vi "Align Traces.vi"(0 "Data Input":T2(array[cluster]) {"Data Channels" format="%.2f"}, 1 "Alignment":enum16{"Vertically", "Horizontally"}(ring)=enum."Horizontally", 3 "Aligning Channel":i32, 4 "Y Level":dbl format="%.2f", 5 "X Level":dbl format="%.2f", 9 "Channels / Subject (in)":T1(array[cluster])=[[{"Start"=0, "End"=1000000, "Offset"=0.0, "Deleted"=FALSE}]] {"Offset" format="%.2f"}) -> (11 "Channels / Subject (out)":T1(array[cluster])=[[{"Start"=0, "End"=1000000, "Offset"=0.0, "Deleted"=FALSE}]] {"Offset" format="%.2f"})   [LabVIEW 2013, in "impulse functions.lvlib"]
uses:
  impulse functions.lvlib
panel:
  # "Copyright Americo A. Migliaccio (c) 2002 All Rights Reserved by Author"
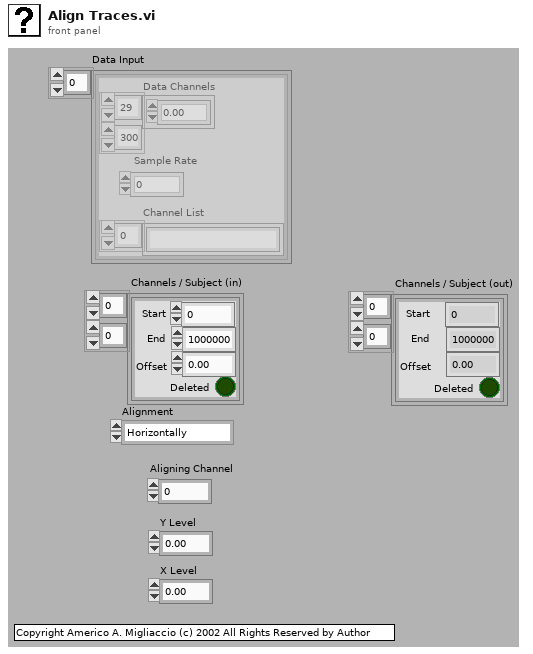
[diagram p1: front panel]
types:
  T1 = cluster{"Start":i32, "End":i32, "Offset":dbl, "Deleted":bool}[][]
  T2 = cluster{"Data Channels":dbl[][], "Sample Rate":i32, "Channel List":string[]}[]
  T3 = cluster{"Start":i32, "End":i32, "Offset":dbl, "Deleted":bool}
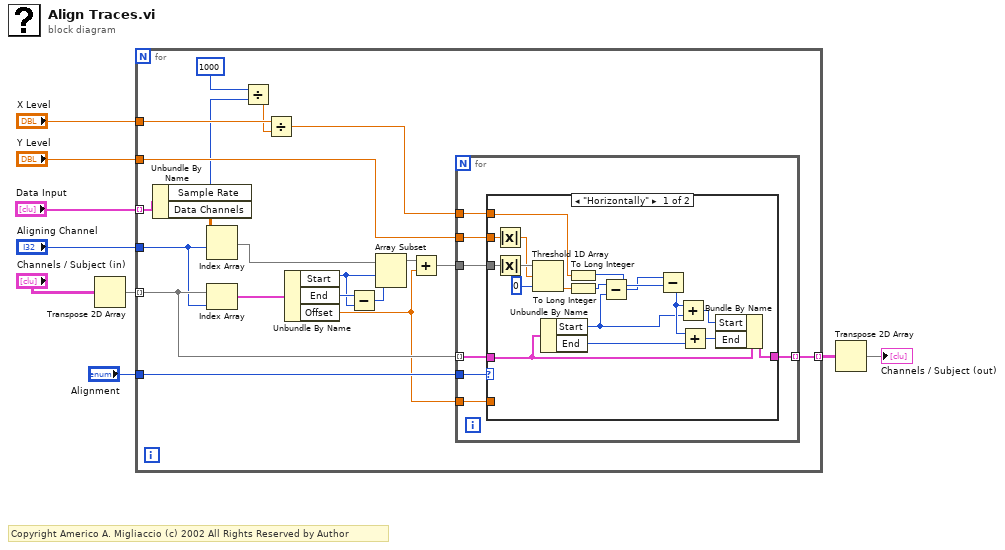
[diagram p0: block diagram]
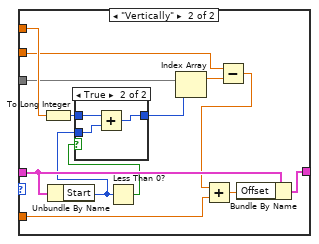
[diagram p2: hidden frame]
diagram:
  # "Copyright Americo A. Migliaccio (c) 2002 All Rights Reserved by Author"
  n1 = Transpose 2D Array(2D array="Channels / Subject (in)") -> (transposed array=w2:T1)
  n2 = for {
    tunnel: "Y Level" -> [w29]
    tunnel: "X Level" -> [w15]
    tunnel: "Alignment" -> [w28]
    tunnel: "Data Input" -> [w27] mode=indexing
    tunnel: "Aligning Channel" -> [w22]
    tunnel: w2 -> [w24] mode=indexing
    tunnel: [w16] -> w3 mode=indexing
    n3 = Unbundle By Name(w27) -> ("Sample Rate"=w14:i32, "Data Channels"=w26:dbl[][])
    n4 = Index Array(array=w26, index (row)=w22) -> (element=w25:dbl[])  [unwired: 1 in]
    n5 = Index Array(array=w24, index=w22) -> (element=w23:T3)
    n6 = Divide(x=1000, y=w14) -> (x/y=w11:dbl)
    n7 = Divide(x=w15, y=w11) -> (x/y=w12:dbl)
    n8 = Unbundle By Name(w23) -> ("Start"=w18:i32, "End"=w19:i32, "Offset"=w10:dbl)
    n9 = Subtract(x=w19, y=w18) -> (x-y=w17:i32)
    n10 = Array Subset(array=w25, index=w18, length=w17) -> (w21:dbl[])
    n11 = Add(x=w21, y=w10) -> (x+y=w20:dbl[])
    n12 = for {
      tunnel: w29 -> [w36]
      tunnel: w12 -> [w35]
      tunnel: w28 -> [w34]
      tunnel: [w33] -> w16 mode=indexing
      tunnel: w20 -> [w32]
      tunnel: w24 -> [w31] mode=indexing
      tunnel: w10 -> [w30]
      n13 = case shown="\"Horizontally\"" w34 {
        tunnel: w31 -> [w45 w63]
        tunnel: w35 -> [w48 w66]
        tunnel: [w46 w64] -> w33
        tunnel: w32 -> [w49 w65]
        tunnel: w36 -> [w52 w62]
        tunnel: w30 -> [_ w54]
        frame "Horizontally" {
          n14 = Absolute Value(x=w52) -> (abs(x)=w50:dbl)
          n15 = Absolute Value(x=w49) -> (abs(x)=w53:dbl[])
          n16 = Threshold 1D Array(1:0 ("start index (0)"), 2:w50, 3:w53) -> (0:w47:dbl)
          n17 = Unbundle By Name(w45) -> ("Start"=w37:i32, "End"=w41:i32)
          n18 = To Long Integer(number=w48) -> (32bit integer=w39:i32)
          n19 = To Long Integer(number=w47) -> (32bit integer=w40:i32)
          n20 = Subtract(x=w40, y=w37) -> (x-y=w38:i32)
          n21 = Subtract(x=w38, y=w39) -> (x-y=w42:i32)
          n22 = Add(x=w42, y=w37) -> (x+y=w44:i32)
          n23 = Add(x=w42, y=w41) -> (x+y=w43:i32)
          n24 = Bundle By Name(cluster=w45, "Start"=w44, "End"=w43) -> (w46:T3)
        }
        frame "Vertically" {
          n25 = To Long Integer(number=w66) -> (32bit integer=w60:i32)
          n26 = Unbundle By Name(w63) -> ("Start"=w55:i32)
          n27 = Less Than 0?(x=w55) -> (x < 0?=w61:bool)
          n28 = case shown="True" w61 {
            tunnel: w60 -> [w67 w70]
            tunnel: [w67 w68] -> w59
            tunnel: w55 -> [_ w69]
            frame False {
            }
            frame True {
              n29 = Add(x=w70, y=w69) -> (x+y=w68:i32)
            }
          }
          n30 = Index Array(array=w65, index=w59) -> (element=w58:dbl)
          n31 = Subtract(x=w62, y=w58) -> (x-y=w56:dbl)
          n32 = Add(x=w56, y=w54) -> (x+y=w57:dbl)
          n33 = Bundle By Name(cluster=w63, "Offset"=w57) -> (w64:T3)
        }
      }
    }
  }
  n34 = Transpose 2D Array(2D array=w3) -> (transposed array=→"Channels / Subject (out)":T1)
